vi "DoRunVInamed.vi"(4 "Scan Period":dbl, 5 "Previous Scan Value":dbl, 6 "Present scan array":dbl[](array[numeric]), 7 "Value to Output":dbl, 8 "Ch Description":T1 {"Duty" format="%016b"; "D" format="%#_5g"; "C" format="%#_5g"; "B" format="%#_5g"; "A" format="%#_5g"}, 9 "Ch names":string[](array[string])) -> (0 "Scan comment":string, 1 "Output":dbl, 3 "HelpText":string="Compares values retrieved from earlier channel with \"map\" of historic values, and warns if new values are out of spec.\nThis help text needs to be made dynamic.\nAcceptable radius (in Y axis units) is in A, minimum number of historic points is in B.")   [LabVIEW 2022 SP3]
uses:
  ADAM Client/Sub VIs/ADAM Controls/Ch_description_ADAM.ctl
  ADAM Client/Sub VIs/ADAM Controls/Module_type_ADAM.ctl
  ADAM Client/Sub VIs/ADAM Controls/Function_ADAM.ctl
  ADAM Client/Sub VIs/ADAM Controls/Channel_State.ctl
  ADAM Client/Sub VIs/ADAM Controls/Calib_type_ADAM.ctl
  ADAM Client/Sub VIs/ADAM Controls/Address.ctl
  <vilib>/Utility/error.llb/Trim Whitespace One-Sided.vi
panel:
  in  "releaseRefs":bool
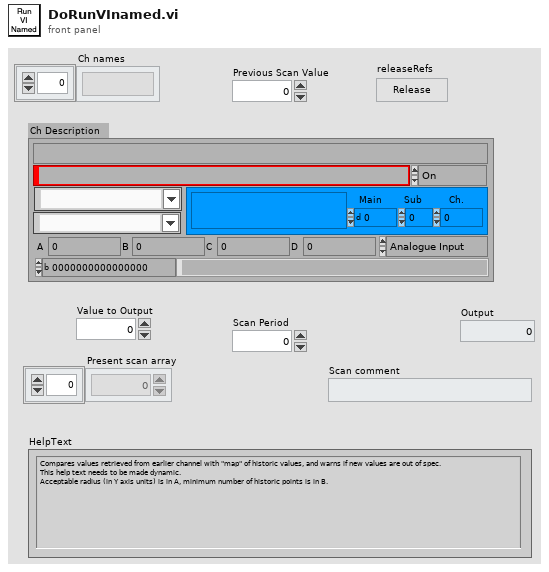
[diagram p1: front panel]
types:
  T1 = typedef "Ch_description_ADAM.ctl" = cluster{"Ch Name":string, "Type":T2, "Function":T3, "Ch State":T4, "Calibration type":T5, "A":dbl, "B":dbl, "C":dbl, "D":dbl, "Comments":string, "Address":T6, "String":string, "Duty":u16}
  T2 = typedef "Module_type_ADAM.ctl" = string
  T3 = typedef "Function_ADAM.ctl" = enum16{"Analogue Input", "Digital Input", "Event counter", "Event rate", "Analogue Output", "Digital Output", "Relay Output"}
  T4 = typedef "Channel_State.ctl" = enum16{"On", "Off", "Always On", "Always Off"}
  T5 = typedef "Calib_type_ADAM.ctl" = string
  T6 = typedef "Address.ctl" = cluster{"Main":i32, "Ch.":i32, "Sub":i32, "Port Name":string}
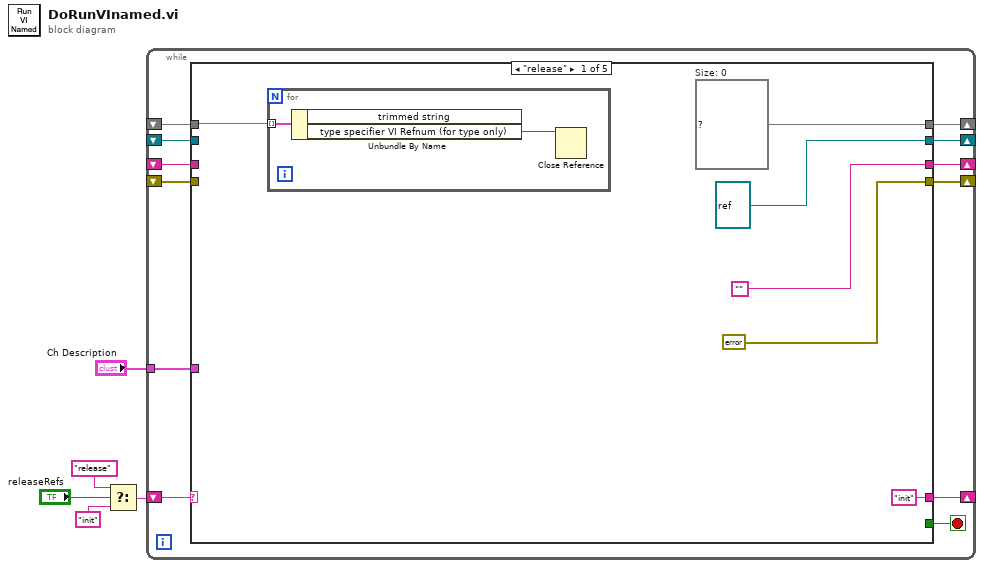
[diagram p0: block diagram]
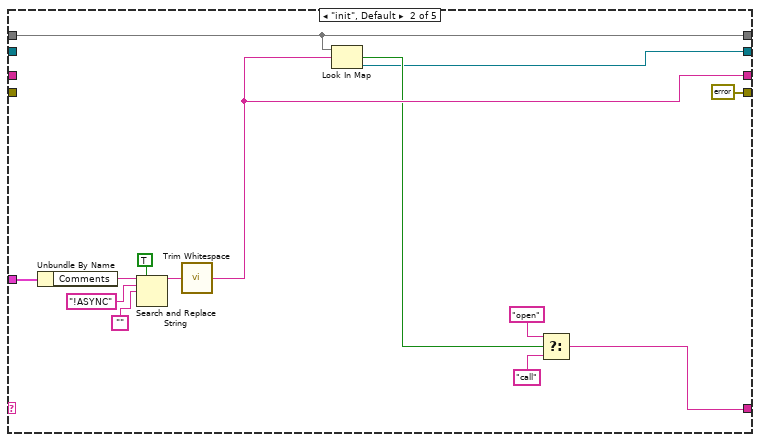
[diagram p2: hidden frame]
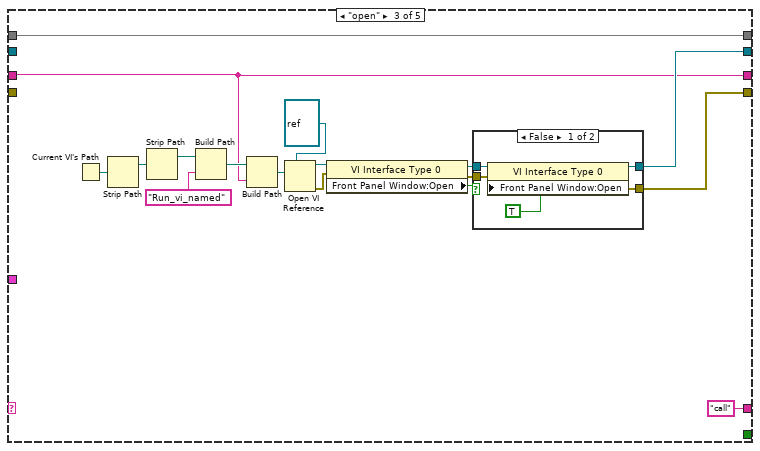
[diagram p3: hidden frame]
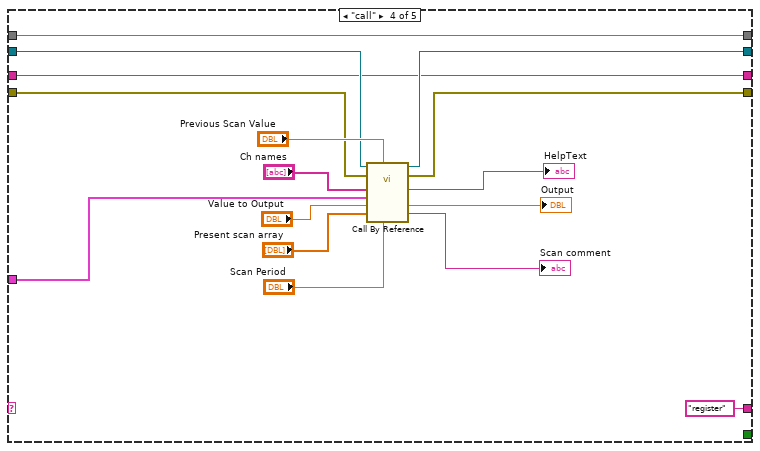
[diagram p5: hidden frame]
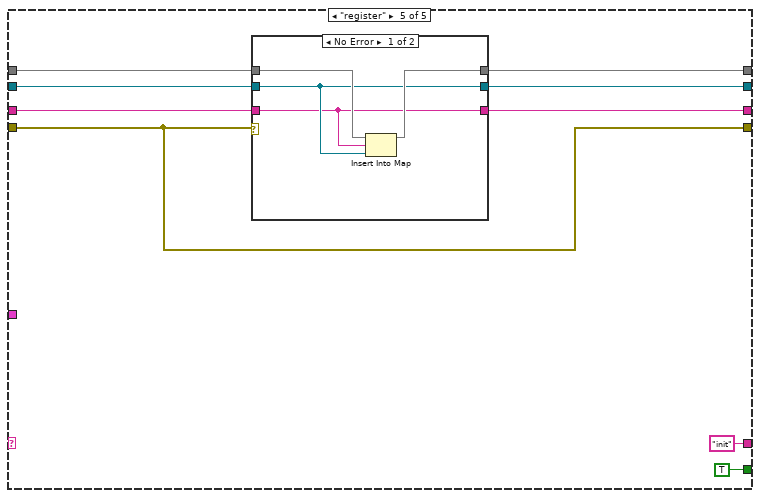
[diagram p6: hidden frame]
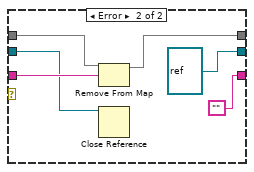
[diagram p7: hidden frame]
diagram:
  n1 = Select(t="release", s="releaseRefs", f="init") -> (s? t:f=w2:string)
  n2 = while {
    shift-right: [w9] -> _
    shift-left: w2 -> [w17]
    tunnel: "Ch Description" -> [w16]
    shift-right: [w12] -> _
    shift-left: _ -> [w15]
    shift-right: [w14] -> _
    shift-left: _ -> [w11]
    shift-right: [w13] -> _
    shift-left: _ -> [w10]
    shift-right: [w8] -> _
    shift-left: _ -> [w7]
    stop <- w6 stop-if-true
    n3 = case shown="\"release\"" w17 {
      tunnel: w16 -> [_ w37 _ w71 _]
      tunnel: w15 -> [w18 w32 w43 w68 w88]
      tunnel: ["" w33 w41 w65 w81] -> w14
      tunnel: [refnum<vi> refnum ("type specifier VI Refnum (for type only)") w27 w44 w67 w82] -> w13
      tunnel: [w23 w32 w43 w68 w87] -> w12
      tunnel: w11 -> [_ _ w41 w65 w86]
      tunnel: w10 -> [_ _ _ w69 w85]
      tunnel: ["init" w30 "call" "register" "init"] -> w9
      tunnel: [errorcluster {"status"=FALSE, "code"=0, "source"=""} ("error out") errorcluster {"status"=FALSE, "code"=0, "source"=""} ("error out") w42 w66 w80] -> w8
      tunnel: w7 -> [_ _ _ w70 w80]
      tunnel: [_ _ _ _ TRUE] -> w6
      frame "release" {
        w23 = map{string, refnum<vi>} {}  # Size: 0
        n4 = for {
          tunnel: w18 -> [w25] mode=indexing
          n5 = Unbundle By Name(w25) -> ("type specifier VI Refnum (for type only)"=w24:refnum<vi>)  [unwired: 1 out]
          n6 = Close Reference(reference=w24) -> ()  [unwired: 1 in, 1 out]
        }
      }
      frame "init", Default {
        n7 = Unbundle By Name(w37) -> ("Comments"=w38:string)
        n8 = Search and Replace String(replace all?=TRUE ("replace all? (F)"), input string=w38, search string="!ASYNC", replace string="") -> (result string=w39:string)  [unwired: 4 in, 3 out]
        n9 = call <vilib>:"Trim Whitespace.vi"("string"=w39) -> ("trimmed string"=w33:string)  [unwired: 1 in]
        n10 = Look In Map(map=w32, key=w33) -> (key not found?=w31:bool, value=w27:refnum<vi>)  [unwired: 1 in]
        n11 = Select(t="open", s=w31, f="call") -> (s? t:f=w30:string)
      }
      frame "open" {
        n12 = Current VI's Path() -> (path=w53:path)
        n13 = Strip Path(path=w53) -> (stripped path=w54:path)  [unwired: 1 out]
        n14 = Strip Path(path=w54) -> (stripped path=w55:path)  [unwired: 1 out]
        n15 = Build Path(base path=w55, name or relative path="Run_vi_named") -> (appended path=w56:path)
        n16 = Build Path(base path=w56, name or relative path=w41) -> (appended path=w52:path)
        n17 = Open VI Reference(type specifier VI Refnum (for type only)=refnum<vi> refnum, vi path=w52) -> (vi reference=w48:refnum<vi>, error out=w47:errorcluster)  [unwired: 1 in, 3 out]
        n18 = property class="VI Interface Type 0"(reference=w48, error in=w47) -> (reference out=w50:refnum<vi>, error out=w49:errorcluster, "Front Panel Window:Open"=w51:bool)
        n19 = case shown="False" w51 {
          tunnel: w50 -> [w61 w63]
          tunnel: w49 -> [w60 w62]
          tunnel: [w59 w63] -> w44
          tunnel: [w57 w62] -> w42
          frame False {
            n20 = property class="VI Interface Type 0"(reference=w61, error in=w60, "Front Panel Window:Open"=TRUE) -> (reference out=w59:refnum<vi>, error out=w57:errorcluster)
          }
          frame True {
          }
        }
      }
      frame "call" {
        n21 = call-by-ref "?"(reference=w69, error in=w70, "Scan Period"="Scan Period", "Previous Scan Value"="Previous Scan Value", "Present scan array"="Present scan array", "Value to Output"="Value to Output", "Ch Description"=w71, "Ch names"="Ch names") -> (reference out=w67:refnum<vi>, error out=w66:errorcluster, "Scan comment"=→"Scan comment":string, "Output"=→"Output":dbl, "HelpText"=→"HelpText":string)  [unwired: 1 in]
      }
      frame "register" {
        n22 = case shown="No Error" w80 {
          tunnel: w88 -> [w92 w98]
          tunnel: [w91 w97] -> w87
          tunnel: w86 -> [w89 w96]
          tunnel: w85 -> [w90 w95]
          tunnel: [w90 refnum<vi> refnum ("type specifier VI Refnum (for type only)")] -> w82
          tunnel: [w89 ""] -> w81
          frame No Error {
            n23 = Insert Into Map(map in=w92, key=w89, value=w90) -> (map out=w91:map{string, refnum<vi>})  [unwired: 2 out]
          }
          frame Error {
            n24 = Remove From Map(10:w96, 11:w98) -> (3:w97:map{string, refnum<vi>})  [unwired: 2 out]
            n25 = Close Reference(reference=w95) -> ()  [unwired: 1 in, 1 out]
          }
        }
      }
    }
  }
